vi "Autosize Tree Row Header Column.vi"(4 "Default Width":u32=50, 6 "Whitespace Border":i16=10, 8 "error in":errorcluster, 9 "reference in":refnum<vi>) -> (0 "error out":errorcluster, 1 "reference out":refnum<vi>)   [LabVIEW 2015]
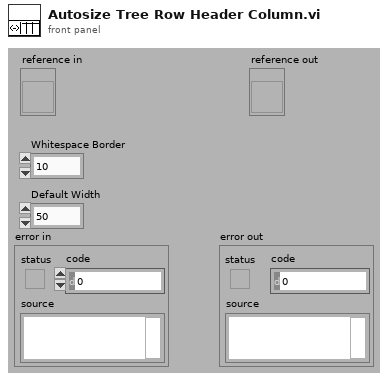
[diagram p1: front panel]
types:
  T1 = enum16{"User-specified Font", "Application Font", "System Font", "Dialog Font"}
  T2 = cluster{"Font Name:":string, "Size":i16, "Strikeout?":bool, "Italic?":bool, "Underline?":bool, "Outline?":bool, "Shadow?":bool, "Bold?":bool}
  T3 = cluster{"left":i16, "top":i16, "right":i16, "bottom":i16}
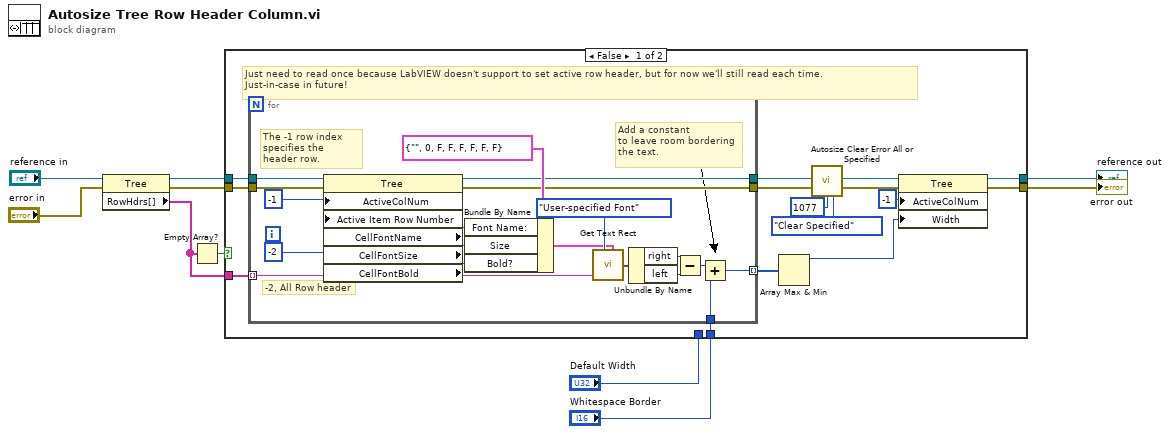
[diagram p0: block diagram]
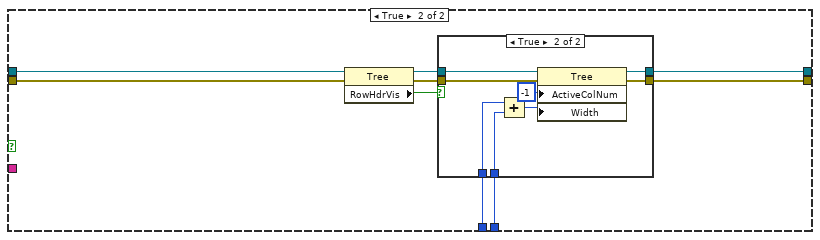
[diagram p2: hidden frame]
diagram:
  n1 = property class="Tree"(reference="reference in", error in="error in") -> (reference out=w5:refnum<vi>, error out=w4:errorcluster, "RowHdrs[]"=w3:string[])
  n2 = Empty Array?(array=w3) -> (empty?=w2:bool)
  n3 = case shown="False" w2 {
    tunnel: w3 -> [w21 _]
    tunnel: w5 -> [w20 w48]
    tunnel: w4 -> [w19 w46]
    tunnel: [w18 w52] -> w8
    tunnel: [w17 w51] -> w9
    tunnel: "Whitespace Border" -> [w16 w49]
    tunnel: "Default Width" -> [_ w50]
    frame False {
      # "Just need to read once because LabVIEW doesn't support to set active row header, but for now we'll still read each time.\nJust-in-case in future!"
      n4 = for {
        tunnel: w20 -> [w43]
        tunnel: [w29] -> w24 mode=indexing
        tunnel: w19 -> [w34]
        tunnel: [w33] -> w12
        tunnel: [w32] -> w23
        tunnel: w16 -> [w28]
        tunnel: w21 -> [w27] mode=indexing
        # "The -1 row index specifies the header row."
        # "Add a constant\nto leave room bordering the text."
        # "-2, All Row header"
        n5 = property class="Tree"(reference=w43, error in=w34, "ActiveColNum"=-1, "Active Item Row Number"=-2 ("Active Item:Row Number")) -> (reference out=w32:refnum<vi>, error out=w33:errorcluster, "CellFontName"=w41:string, "CellFontSize"=w30:u32, "CellFontBold"=w40:bool)
        n6 = Bundle By Name(cluster=T2 {"Font Name:"="", "Size"=0, "Strikeout?"=FALSE, "Italic?"=FALSE, "Underline?"=FALSE, "Outline?"=FALSE, "Shadow?"=FALSE, "Bold?"=FALSE} ("[user-specified font]"), "Font Name:"=w41, "Size"=w30, "Bold?"=w40) -> (w38:T2)
        n7 = call <vilib>:"Get Text Rect.vi"("desired font(Application)"=T1."User-specified Font", "text"=w27, "[user-specified font]"=w38) -> ("rect"=w37:T3)  [unwired: 3 in, 3 out]
        n8 = Unbundle By Name(w37) -> ("right"=w36:i16, "left"=w35:i16)
        n9 = Subtract(x=w36, y=w35) -> (x-y=w31:i16)
        n10 = Add(x=w31, y=w28) -> (x+y=w29:i16)
      }
      n11 = Array Max & Min(array=w24) -> (max value=w22:i16)  [unwired: 3 out]
      n12 = call "Autosize Clear Error All or Specified.vi"("Clear Mode (0: Clear All)"=enum16{"Clear All", "Clear Specified"}."Clear Specified", "Code to Clear (0)"=1077 ("[exception code]"), "error in (no error)"=w12) -> ("error out"=w11:errorcluster)  [unwired: 1 in, 11 out]
      n13 = property class="Tree"(reference=w23, error in=w11, "ActiveColNum"=-1, "Width"=w22) -> (reference out=w18:refnum<vi>, error out=w17:errorcluster)
    }
    frame True {
      n14 = property class="Tree"(reference=w48, error in=w46) -> (reference out=w47:refnum<vi>, error out=w45:errorcluster, "RowHdrVis"=w44:bool)
      n15 = case shown="True" w44 {
        tunnel: [w54 w62] -> w52
        tunnel: [w53 w61] -> w51
        tunnel: w50 -> [_ w60]
        tunnel: w49 -> [_ w59]
        tunnel: w47 -> [w54 w57]
        tunnel: w45 -> [w53 w56]
        frame False {
          # "Don't care..!"
        }
        frame True {
          n16 = Add(x=w60, y=w59) -> (x+y=w58:u32)
          n17 = property class="Tree"(reference=w57, error in=w56, "ActiveColNum"=-1, "Width"=w58) -> (reference out=w62:refnum<vi>, error out=w61:errorcluster)
        }
      }
    }
  }
  "error out" <- w9
  "reference out" <- w8
